vi "HandleRemoteMessage.vi"(6 "driver status":T1, 8 "error in (no error)":errorcluster, 9 "Message data":variant, 10 "Sender":string, 11 "RemoteConnection in":refnum<class "RemoteConnection.lvclass">) -> (0 "error out":errorcluster, 3 "RemoteConnection out":refnum<class "RemoteConnection.lvclass">)   [LabVIEW 2013, in "RemoteConnection.lvclass"]
uses:
  RemoteConnection.lvclass
  driver_status.ctl
  TcpDriver/MixerResponse.ctl
  Message/MixerMessage/MixerOperation.ctl
  Message/MixerMessage/MixerParam.ctl
  RemoteConnection.lvclass/RemoteConnection.ctl
  message_queue.ctl
  Message/BaseMessage/BaseMessage.lvclass
  Message/MixerMessage/MixerMessage.lvclass
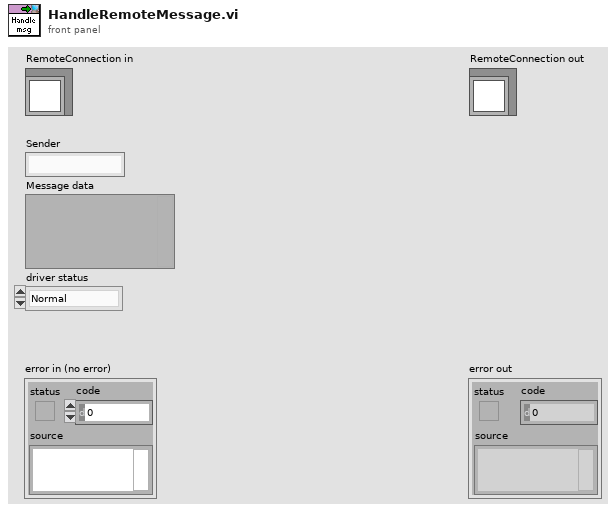
[diagram p1: front panel]
types:
  T1 = typedef "driver_status.ctl" = enum16{"Normal", "Startup", "Connection lost", "Reconnected", "Timeout", "Idle", "Busy"}
  T2 = typedef "MixerResponse.ctl" = cluster{"Operation":T3, "Param":T4, "value":dbl}
  T3 = typedef "MixerMessage.lvclass/MixerOperation.ctl" = enum16{"Get", "Set"}
  T4 = typedef "MixerMessage.lvclass/MixerParam.ctl" = enum16{"a", "b", "fm"}
  T5 = typedef "message_queue.ctl" = refnum<queue>
  T6 = typedef "RemoteConnection.lvclass/RemoteReferences.ctl" = cluster{"a":refnum<vi>, "b":refnum<vi>, "fm":refnum<vi>}
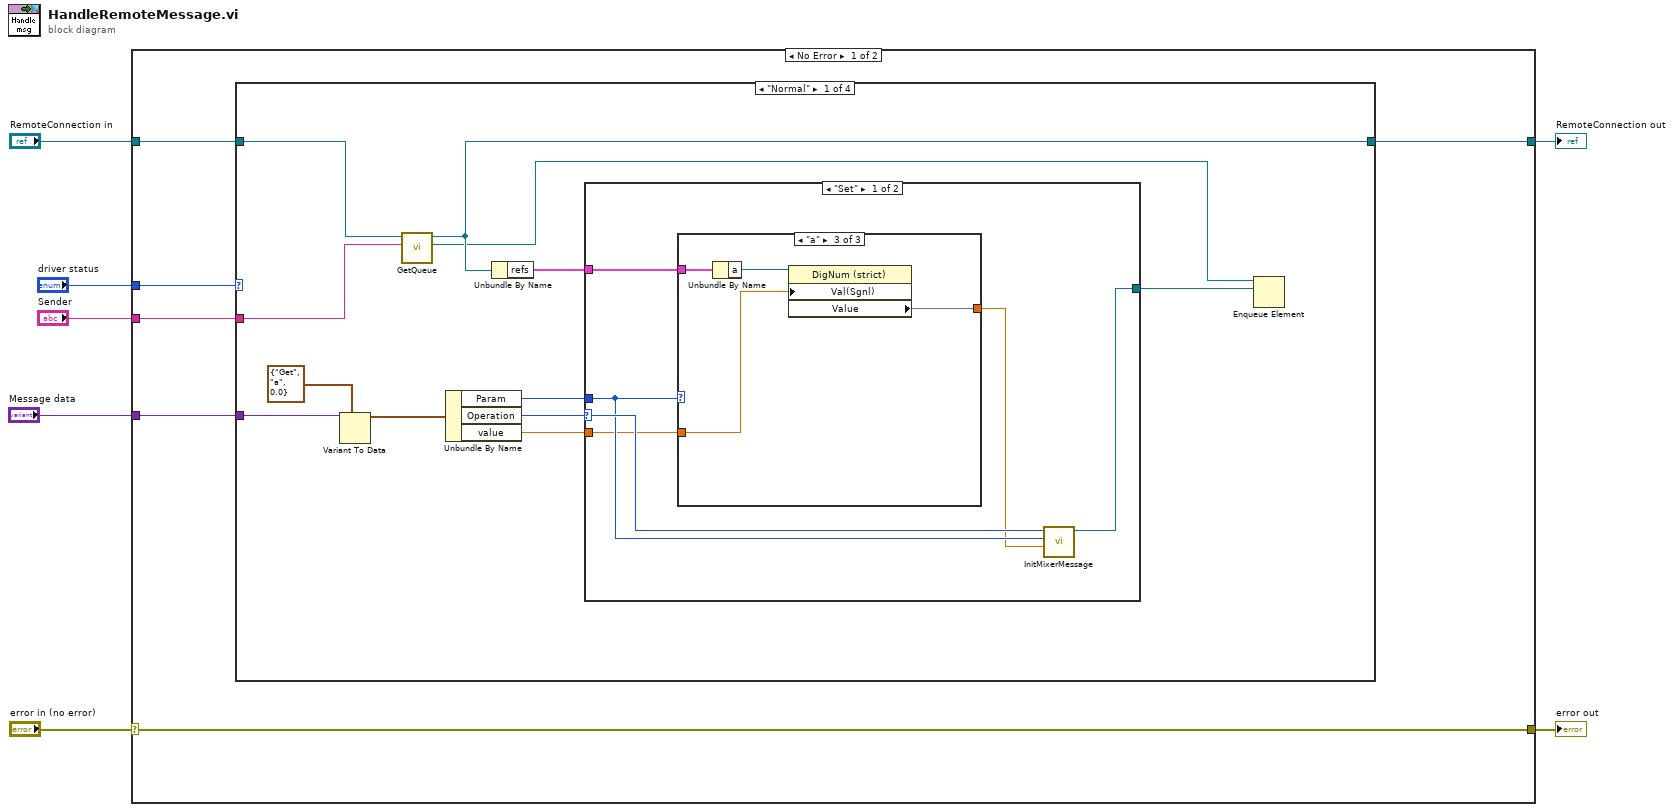
[diagram p0: block diagram]
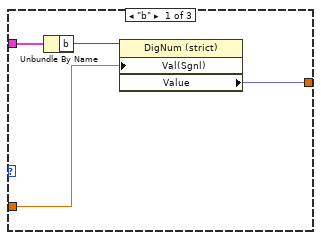
[diagram p2: hidden frame]
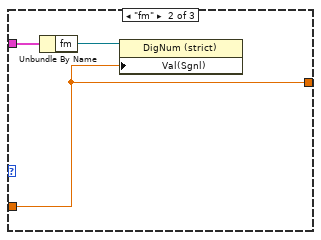
[diagram p3: hidden frame]
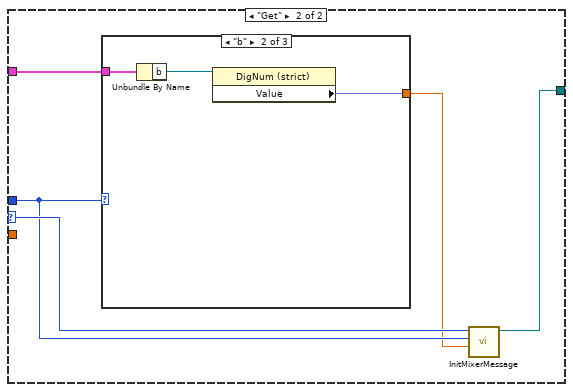
[diagram p4: hidden frame]
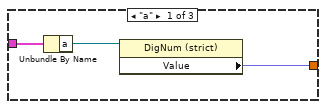
[diagram p5: hidden frame]
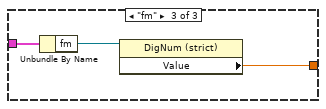
[diagram p6: hidden frame]
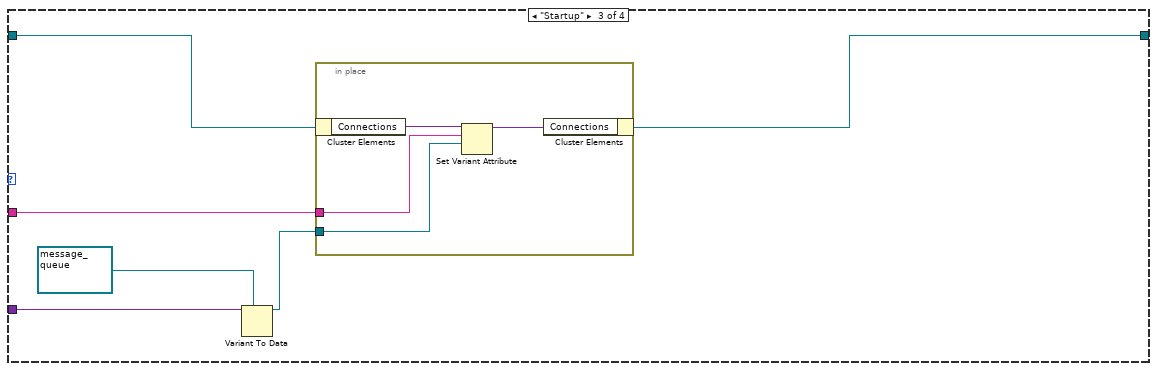
[diagram p8: hidden frame]
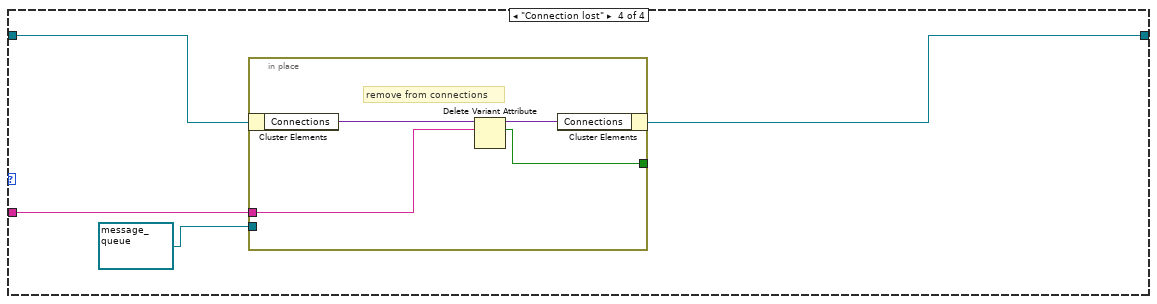
[diagram p9: hidden frame]
diagram:
  n1 = case shown="No Error" "error in (no error)" {
    selector: "error in (no error)" -> [w13 w77]
    tunnel: [w13 w77] -> w6
    tunnel: [w9 w76] -> w4
    tunnel: "RemoteConnection in" -> [w10 w76]
    tunnel: "driver status" -> [w12 _]
    tunnel: "Message data" -> [w11 _]
    tunnel: "Sender" -> [w8 _]
    frame No Error {
      n2 = case shown="\"Normal\"" w12 {
        tunnel: w11 -> [w25 _ w63 _]
        tunnel: w10 -> [w23 w57 w61 w71]
        tunnel: [w20 w57 w58 w68] -> w9
        tunnel: w8 -> [w22 _ w60 w70]
        frame "Normal" {
          n3 = Variant To Data(type=T2 {"Operation"=enum."Get", "Param"=enum."a", "value"=0.0} ("MixerRespone"), Variant=w25) -> (data=w21:T2)  [unwired: 1 in, 1 out]
          n4 = call "GetQueue.vi"("Sender"=w22, "RemoteConnection In"=w23) -> ("Queue"=w15:T5, "RemoteConnection Out"=w20:refnum<class "RemoteConnection.lvclass">)  [unwired: 7 in, 1 out]
          n5 = Unbundle By Name(w21) -> ("Param"=w17:T4, "Operation"=w18:T3, "value"=w16:dbl)
          n6 = Unbundle By Name(w20) -> ("refs"=w19:T6)
          n7 = case shown="\"Set\"" w18 {
            selector: w18 -> [w30 w46]
            tunnel: w19 -> [w31 w47]
            tunnel: w17 -> [w29 w45]
            tunnel: w16 -> [w28 _]
            tunnel: [w27 w44] -> w14
            frame "Set" {
              n8 = case shown="\"a\"" w29 {
                tunnel: w28 -> [w33 w36 w40]
                tunnel: w31 -> [w35 w38 w42]
                tunnel: [w32 w36 w39] -> w26
                frame "b" {
                  n9 = Unbundle By Name(w35) -> ("b"=w34:refnum<vi>)
                  n10 = property class="DigNum (strict)"(reference=w34, "Val(Sgnl)"=w33) -> ("Value"=w32:fxp<+/-,16,2>)  [unwired: 1 in, 2 out]
                }
                frame "fm" {
                  n11 = Unbundle By Name(w38) -> ("fm"=w37:refnum<vi>)
                  n12 = property class="DigNum (strict)"(reference=w37, "Val(Sgnl)"=w36) -> ()  [unwired: 1 in, 2 out]
                }
                frame "a" {
                  n13 = Unbundle By Name(w42) -> ("a"=w41:refnum<vi>)
                  n14 = property class="DigNum (strict)"(reference=w41, "Val(Sgnl)"=w40) -> ("Value"=w39:fxp<+/-,16,2>)  [unwired: 1 in, 2 out]
                }
              }
              n15 = call "InitMixerMessage.vi"("value"=w26, "Param"=w29, "Operation"=w30) -> ("MixerMessage out"=w27:refnum<class "MixerMessage.lvclass">)  [unwired: 8 in]
            }
            frame "Get" {
              n16 = case shown="\"b\"" w45 {
                tunnel: w47 -> [w50 w53 w56]
                tunnel: [w48 w51 w54] -> w43
                frame "a" {
                  n17 = Unbundle By Name(w50) -> ("a"=w49:refnum<vi>)
                  n18 = property class="DigNum (strict)"(reference=w49) -> ("Value"=w48:fxp<+/-,16,2>)  [unwired: 1 in, 2 out]
                }
                frame "b" {
                  n19 = Unbundle By Name(w53) -> ("b"=w52:refnum<vi>)
                  n20 = property class="DigNum (strict)"(reference=w52) -> ("Value"=w51:fxp<+/-,16,2>)  [unwired: 1 in, 2 out]
                }
                frame "fm" {
                  n21 = Unbundle By Name(w56) -> ("fm"=w55:refnum<vi>)
                  n22 = property class="DigNum (strict)"(reference=w55) -> ("Value"=w54:dbl)  [unwired: 1 in, 2 out]
                }
              }
              n23 = call "InitMixerMessage.vi"("value"=w43, "Param"=w45, "Operation"=w46) -> ("MixerMessage out"=w44:refnum<class "MixerMessage.lvclass">)  [unwired: 8 in]
            }
          }
          n24 = Enqueue Element(queue=w15, element=w14) -> ()  [unwired: 2 in, 3 out]
        }
        frame Default {
        }
        frame "Startup" {
          n25 = Variant To Data(type=T5 refnum ("Input queue"), Variant=w63) -> (data=w59:T5)  [unwired: 1 in, 1 out]
          n26 = in-place {
            in-place-border: w60 -> [w66]
            in-place-border: w59 -> [w65]
            n27 = in-place-cluster #1(w61) -> ("Connections"=w67:variant)
            n28 = Set Variant Attribute(Variant=w67, name=w66, value=w65) -> (Variant out=w64:variant)  [unwired: 1 in, 2 out]
            n29 = in-place-cluster #1("Connections"=w64) -> (w58:refnum<class "RemoteConnection.lvclass">)
          }
        }
        frame "Connection lost" {
          n30 = in-place {
            in-place-border: w70 -> [w74]
            in-place-border: T5 refnum ("Input queue") -> [_]
            in-place-border: [w73] -> _
            # "remove from connections"
            n31 = in-place-cluster #2(w71) -> ("Connections"=w72:variant)
            n32 = Delete Variant Attribute(6:w74, 7:w72) -> (2:w73:bool, 3:w75:variant)  [unwired: 1 in, 1 out]
            n33 = in-place-cluster #2("Connections"=w75) -> (w68:refnum<class "RemoteConnection.lvclass">)
          }
        }
      }
    }
    frame Error {
    }
  }
  "error out" <- w6
  "RemoteConnection out" <- w4
